vi "Save Digital Data.vi"(8 "error in (no error)":errorcluster, 10 "Data Cluster":cluster{"Path":path, "Array":bool[]}, 11 "Digital TDMS in":refnum<class "Digital TDMS.lvclass">) -> (0 "error out":errorcluster, 3 "Digital TDMS out":refnum<class "Digital TDMS.lvclass">)   [LabVIEW 2020, in "Digital TDMS.lvlib" / "Digital TDMS.lvclass"]
uses:
  Digital TDMS.lvclass
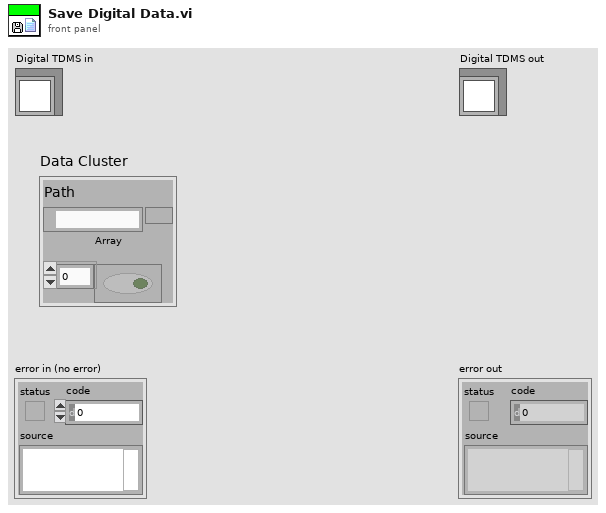
[diagram p1: front panel]
types:
  T1 = enum16{"open", "open or create", "create or replace", "create", "open (read-only)"}
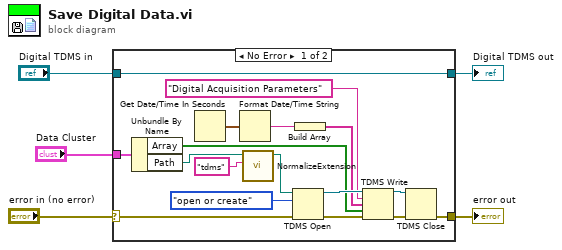
[diagram p0: block diagram]
diagram:
  n1 = case shown="No Error" "error in (no error)" {
    selector: "error in (no error)" -> [w20 w23]
    tunnel: "Digital TDMS in" -> [w22 w24]
    tunnel: [w22 w24] -> w1
    tunnel: [w9 w23] -> w2
    tunnel: "Data Cluster" -> [w8 _]
    frame No Error {
      n2 = Unbundle By Name(w8) -> ("Array"=w6:bool[], "Path"=w7:path)
      n3 = Get Date/Time In Seconds() -> (seconds since 1Jan1904=w14:timestamp)
      n4 = Format Date/Time String(seconds (now)=w14) -> (date/time string=w13:string)  [unwired: 2 in]
      n5 = call "NormalizeExtension.vi"("Extension"="tdms", "Path in"=w7) -> ("Path out"=w19:path)  [unwired: 9 in]
      n6 = TDMS Open(8:w20, 10:T1."open or create" ("operation (0:open)"), 11:w19) -> (0:w16:errorcluster, 3:w17:refnum<k34>)  [unwired: 4 in]
      n7 = Build Array(w13) -> (w12:string[])
      n8 = TDMS Write(0:w17, 5:"Digital Acquisition Parameters" ("group name in (Untitled)"), 7:w12, 9:w6, 11:w16) -> (4:w10:refnum<k34>, 15:w11:errorcluster)  [unwired: 1 in, 2 out]
      n9 = TDMS Close(8:w11, 11:w10) -> (0:w9:errorcluster)  [unwired: 1 out]
    }
    frame Error {
    }
  }
  "error out" <- w2
  "Digital TDMS out" <- w1
